vi "Log_Add.vi"(3 "Log":string) -> ()   [LabVIEW 2015]
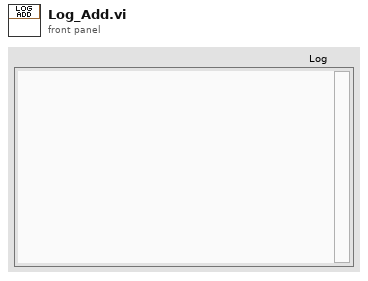
[diagram p1: front panel]
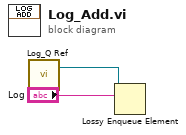
[diagram p0: block diagram]
diagram:
  n1 = call "Log_Q Ref.vi"() -> ("Log Queue"=w2:refnum<queue>)  [unwired: 3 in]
  n2 = Lossy Enqueue Element(queue=w2, element="Log") -> ()  [unwired: 1 in, 4 out]
